vi "SLL Error Simulation Global.vi"() -> ()   [LabVIEW 2013]
doc: "Copyright © 2007, Soliton Technologies. All rights reserved."
panel:
  in  "Error Descriptions":string[](array[string])
  in  "Error Codes":string[](array[string])
  in  "Cases":string[](array[string])
  in  "Caller":string[](array[string])
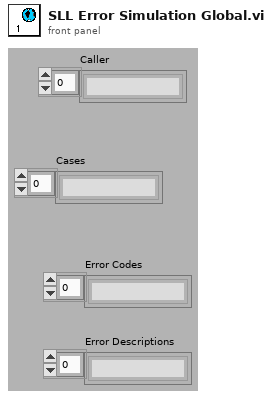
[diagram p1: front panel]
diagram:
